vi "set_in_plane_move_speeds_Z-tilt.vi"(6 "Z tilt (angle)":dbl, 7 "Use standard V_max (t)":bool=TRUE, 8 "error in (no error)":errorcluster, 10 "V_max Z":dbl=15000.0, 11 "VISA resource name":refnum<visa-resource-name>) -> (0 "error out":errorcluster={"status"=FALSE, "code"=1073676294, "source"="VISA Read in write_read.vi"}, 1 "V_max Motor 2":i32, 2 "V_max Motor 3":i32, 3 "VISA ressource out":refnum<visa-resource-name>)   [LabVIEW 2018]
uses:
  MCode_LV_86/Set Parameter.ctl
  ConversionAndInformation/Unit_Control.ctl
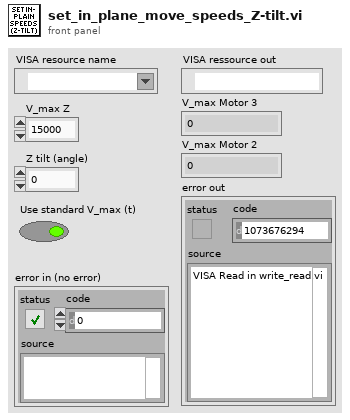
[diagram p1: front panel]
types:
  T1 = typedef "Unit_Control.ctl" = enum16{"Angle (Degrees)", "Rad", "Angle [TMC]", "Microsteps [TMC]", "Inches", "Nanometer", "Meter", "Centimeter", "Millimeter", "Micron"}
  T2 = typedef "Set Parameter.ctl" = enum16{"Acceleration (A)", "Baud Rate (BD)", "Counter 1 (C1)", "Counter 2 (C2)", "Control C Software Reset (CE)", "Check Sum Enable (CK)", "Clock Mode (CM)", "Clock Mode Ratio (CR)", "Clock Mode Out Step Width (CW)", "Deceleration (D)", "Digital Filtering, Input 1 (D1)", "Digital Filtering, Input 2 (D2)", "Digital Filtering, Input 3 (D3)", "Digital Filtering, Input 4 (D4)", "Digital Filtering, Input 5 (D5)", "Digital Filtering, Input 9 (D9)", "Digital Filtering, Input 10 (D10)", "Digital Filtering, Input 11 (D11)", "Digital Filtering, Input 12 (D12)", "Deadband (DB)", "Decrement Variable (DC)", "Enable/Disable Drive (DE)", "Device Name (DN)", "End Program Execution (E)", "Encoder Function Enable (EE)", "Error Flag (EF)", "Encoder Lines (EL)", "Echo Mode (EM)", "Error Value (ER)", "Escape (ES)", "Execute Program at Address (EX)", "Firmware Version (VR)", "Hold (H)", "Hold Current (HC)", "Hold Current Delay Time (HI)", "Home to Encoder Index (HM)", "Home to Home Switch (HT)", "Increment Variable (IC)", "Initialize Parameters to NVM (IP)", "Input into Variable (IV)", "Jog Enable (JE)", "Limit Stop Mode (LM)", "Move Absolute (MA)", "Move Relative (MR)", "MicroStepping Select (MS)", "Motor Settling Delay Time (MT)", "Moving [Flag] (MV)", "Output 1 (O1)", "Output 2 (O2)", "Output 3 (O3)", "Output 4 (O4)", "Output 9 (O9)", "Output 10 (O10)", "Output 11 (O11)", "Output 12 (O12)", "Output High Byte (9-12) (OH)", "Output Low Byte (1-4) (OL)", "Output Total (1-4 and 9-12) (OT)", "Position (P)", "Position Maintenance (PM)", "Party Mode (PY)", "Register 1 (R1)", "Register 2 (R2)", "Register 3 (R3)", "Register 4 (R4)", "Reset Error(\\03)", "Run Current (RC)", "Stall Factor (SF)", "Slew (SL)", "Stall Mode Set (SM)", "Upgrade Firmware (UG)", "Velocity Initial (VI)", "Velocity Maximum (VM)", "Current1 (I1)", "Current2 (I2)", "Current3 (I3)", "Current4 (I4)", "Current5 (I5)", "Current6 (I6)", "Save (S)"}
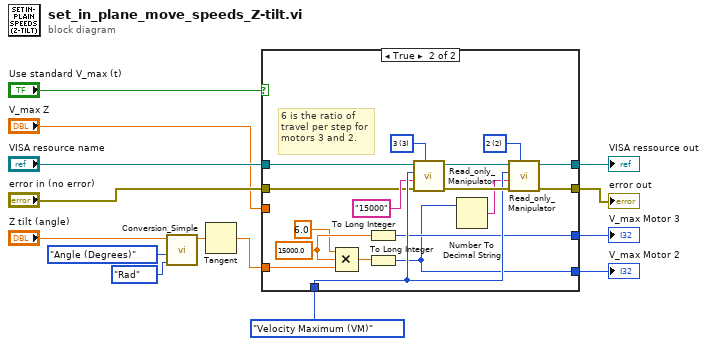
[diagram p0: block diagram]
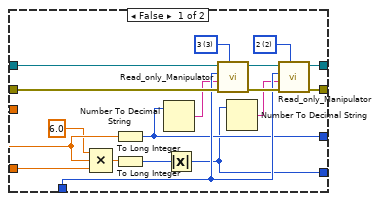
[diagram p2: hidden frame]
diagram:
  n1 = call "Conversion_Simple.vi"("Output Unit"=Unit_Control."Rad", "Input Unit"=Unit_Control."Angle (Degrees)", "Input"="Z tilt (angle)") -> ("Output"=w4:dbl)  [unwired: 7 in, 1 out]
  n2 = Tangent(1:w4) -> (0:w1:dbl)
  n3 = case shown="True" "Use standard V_max (t)" {
    tunnel: [w28 w45] -> w14
    tunnel: [w27 w43] -> w13
    tunnel: "V_max Z" -> [w21 _]
    tunnel: [w20 w36] -> w12
    tunnel: [w16 w35] -> w11
    tunnel: "VISA resource name" -> [w26 w46]
    tunnel: "error in (no error)" -> [w25 w40]
    tunnel: Set_Parameter."Velocity Maximum (VM)" ("Command") -> [w24 w42]
    tunnel: w1 -> [w22 w39]
    frame False {
      w30 = u16 3 items=["none", "1", "2", "3", "4", "all"] ("Motor")
      w29 = u16 2 items=["none", "1", "2", "3", "4", "all"] ("Motor")
      n4 = Compound Arithmetic op=MULTIPLY(6.0, w21, w22) -> (w23:dbl)
      n5 = To Long Integer(number=w21) -> (32bit integer=w20:i32)
      n6 = To Long Integer(number=w23) -> (32bit integer=w17:i32)
      n7 = Number To Decimal String(number=w20) -> (decimal integer string=w19:string)  [unwired: 1 in]
      n8 = Absolute Value(x=w17) -> (abs(x)=w16:i32)
      n9 = call "Read_only_Manipulator.vi"("Motor"=w30, "error in (no error)"=w25, "Value"=w19, "Command"=w24, "VISA resource name"=w26) -> ("error out"=w32:errorcluster, "VISA ressource out"=w31:refnum<visa-resource-name>)  [unwired: 3 in, 2 out]
      n10 = Number To Decimal String(number=w16) -> (decimal integer string=w18:string)  [unwired: 1 in]
      n11 = call "Read_only_Manipulator.vi"("Motor"=w29, "error in (no error)"=w32, "Value"=w18, "Command"=w24, "VISA resource name"=w31) -> ("error out"=w27:errorcluster, "VISA ressource out"=w28:refnum<visa-resource-name>)  [unwired: 3 in, 2 out]
    }
    frame True {
      w37 = 15000.0
      w48 = u16 3 items=["none", "1", "2", "3", "4", "all"] ("Motor")
      w47 = u16 2 items=["none", "1", "2", "3", "4", "all"] ("Motor")
      # "6 is the ratio of\ntravel per step for\nmotors 3 and 2."
      n12 = Compound Arithmetic op=MULTIPLY(6.0, w37, w39) -> (w38:dbl)
      n13 = To Long Integer(number=w37) -> (32bit integer=w36:i32)
      n14 = To Long Integer(number=w38) -> (32bit integer=w35:i32)
      n15 = call "Read_only_Manipulator.vi"("Motor"=w48, "error in (no error)"=w40, "Value"="15000", "Command"=w42, "VISA resource name"=w46) -> ("error out"=w44:errorcluster, "VISA ressource out"=w49:refnum<visa-resource-name>)  [unwired: 3 in, 2 out]
      n16 = Number To Decimal String(number=w35) -> (decimal integer string=w34:string)  [unwired: 1 in]
      n17 = call "Read_only_Manipulator.vi"("Motor"=w47, "error in (no error)"=w44, "Value"=w34, "Command"=w42, "VISA resource name"=w49) -> ("error out"=w43:errorcluster, "VISA ressource out"=w45:refnum<visa-resource-name>)  [unwired: 3 in, 2 out]
    }
  }
  "VISA ressource out" <- w14
  "error out" <- w13
  "V_max Motor 3" <- w12
  "V_max Motor 2" <- w11
